vi "Activate-combined-measurement-hardware.vi"(8 "error in (no error)":errorcluster, 11 "SM1000-control in":T1) -> (0 "error out":errorcluster, 1 "Signals":refnum<k21>, 2 "Control":refnum<k21>, 3 "SM1000-control out":T1, 4 "Batch size":i32)   [LabVIEW 2013, in "MaterialCharacterization.lvlib" / "MC-SM1000.lvclass"]
uses:
  MC-SM1000.lvclass
  Object-reference.ctl
  MC-SM1000.lvclass/MC-SM1000.ctl
  <vilib>/DAQmx/create/channels.llb/DAQmx Create Channel (DI-Digital Input).vi
  <vilib>/DAQmx/configure/timing.llb/DAQmx Timing (Sample Clock).vi
  <vilib>/DAQmx/create/channels.llb/DAQmx Create Channel (AI-Temperature-Thermocouple).vi
  <vilib>/DAQmx/create/channels.llb/DAQmx Create Channel (AI-Voltage-Basic).vi
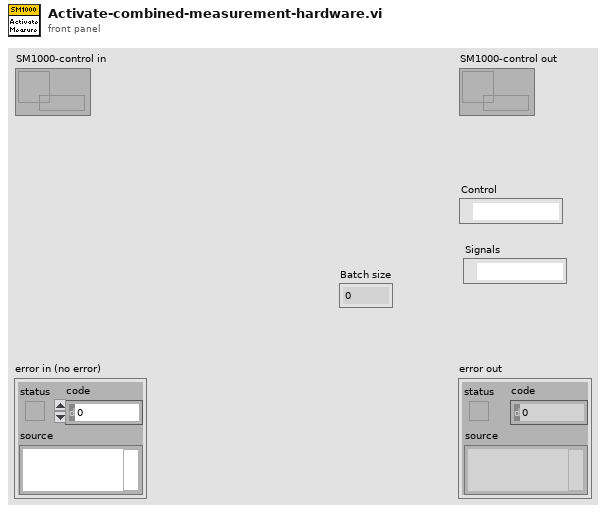
[diagram p1: front panel]
types:
  T1 = typedef "MaterialCharacterization.lvlib/MC-SM1000.lvclass/Object-reference.ctl" = refnum<data-value>
  T2 = typedef "MaterialCharacterization.lvlib/MC-SM1000.lvclass/Combined-settings.ctl" = cluster{"Sample rate":dbl, "Batch size":i32, "Modulation channel":tag, "Temperature channel":tag, "Reflection channel":tag, "Power channel":tag}
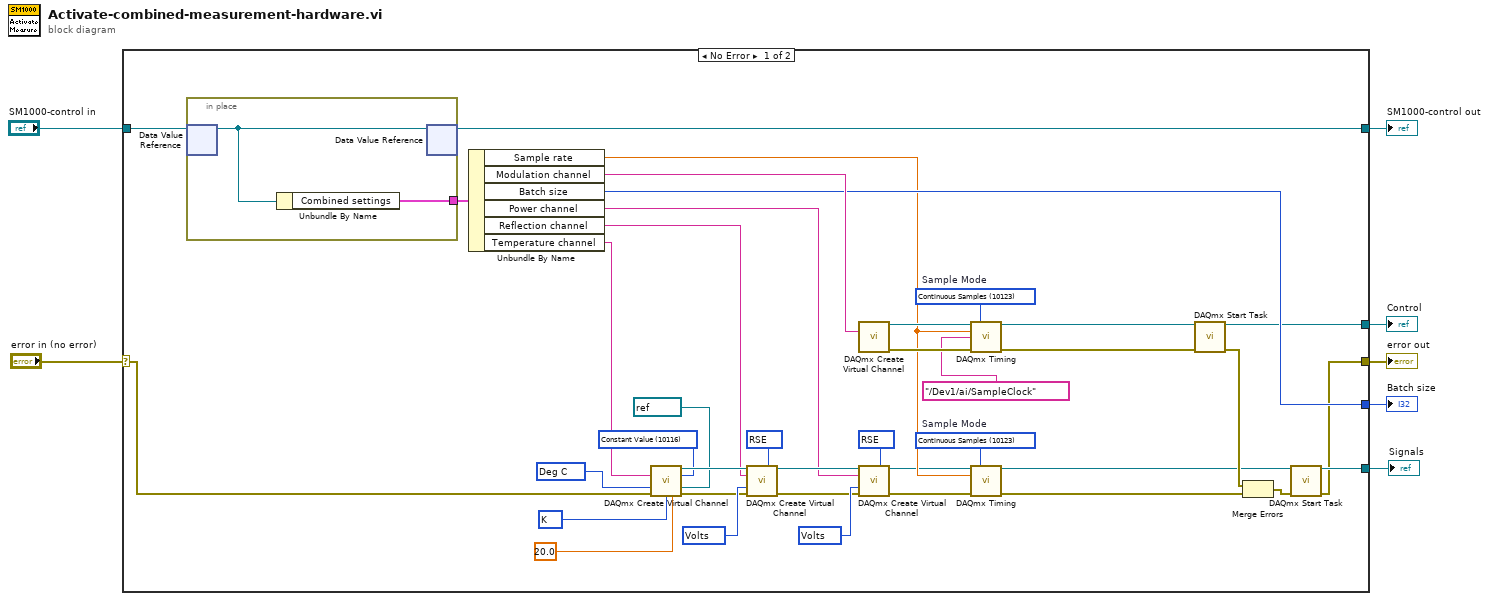
[diagram p0: block diagram]
diagram:
  n1 = case shown="No Error" "error in (no error)" {
    selector: "error in (no error)" -> [w16 w50]
    tunnel: [w32 w50] -> w6
    tunnel: [w45 w49] -> w4
    tunnel: "SM1000-control in" -> [w46 w49]
    tunnel: [w31 _] -> w3
    tunnel: [w39 _] -> w2
    tunnel: [w35 _] -> w1
    frame No Error {
      w11 = 10143 items=["Deg C"=10143, "Deg F"=10144, "Kelvins"=10325, "Deg R"=10145, "From Custom Scale"=10065] ("units")
      w13 = 10116 items=["Built-In"=10200, "Constant Value"=10116, "Channel"=10113] ("cjc source")
      w15 = 10073 items=["J"=10072, "K"=10073, "N"=10077, "R"=10082, "S"=10085, "T"=10086, "B"=10047, "E"=10055] ("thermocouple type")
      w25 = 10348 items=["Volts"=10348, "From Custom Scale"=10065] ("units")
      w24 = 10083 items=["default"=-1, "RSE"=10083, "NRSE"=10078, "Differential"=10106, "Pseudodifferential"=12529] ("input terminal configuration")
      w36 = 10348 items=["Volts"=10348, "From Custom Scale"=10065] ("units")
      w37 = 10083 items=["default"=-1, "RSE"=10083, "NRSE"=10078, "Differential"=10106, "Pseudodifferential"=12529] ("input terminal configuration")
      w38 = 10123 items=["Finite Samples"=10178, "Continuous Samples"=10123, "Hardware Timed Single Point"=12522]  # Sample Mode
      w43 = 10123 items=["Finite Samples"=10178, "Continuous Samples"=10123, "Hardware Timed Single Point"=12522]  # Sample Mode
      n2 = in-place {
        in-place-border: [w47] -> w44
        n3 = in-place-dvr #1(w46) -> (w48:refnum<class "MC-SM1000.lvclass">)  [unwired: 1 out]
        n4 = Unbundle By Name(w48) -> ("Combined settings"=w47:T2)
        n5 = in-place-dvr #1(w48) -> (w45:T1)  [unwired: 1 out]
      }
      n6 = Unbundle By Name(w44) -> ("Sample rate"=w26:dbl, "Modulation channel"=w40:tag, "Batch size"=w39:i32, "Power channel"=w9:tag, "Reflection channel"=w10:tag, "Temperature channel"=w12:tag)
      n7 = call-poly <vilib>:"DAQmx Create Virtual Channel.vi"("physical channels"=w12, "cjc source"=w13, "units"=w11, "cjc channel"=refnum<k21> "CJC", "error in"=w16, "thermocouple type"=w15, "cjc value"=20.0) -> ("task out"=w18:refnum<k21>, "error out"=w17:errorcluster)  [unwired: 7 in]
      n8 = call-poly <vilib>:"DAQmx Create Virtual Channel.vi"("task in"=w18, "input terminal configuration"=w37, "physical channels"=w10, "units"=w36, "error in"=w17) -> ("task out"=w23:refnum<k21>, "error out"=w19:errorcluster)  [unwired: 9 in]
      n9 = call-poly <vilib>:"DAQmx Create Virtual Channel.vi"("lines"=w40) -> ("task out"=w42:refnum<k21>, "error out"=w41:errorcluster)  [unwired: 13 in]
      n10 = call-poly <vilib>:"DAQmx Create Virtual Channel.vi"("task in"=w23, "input terminal configuration"=w24, "physical channels"=w9, "units"=w25, "error in"=w19) -> ("task out"=w22:refnum<k21>, "error out"=w21:errorcluster)  [unwired: 9 in]
      n11 = call-poly <vilib>:"DAQmx Timing.vi"("task/channels in"=w42, "sample mode"=w43, "rate"=w26, "source"=tag "/Dev1/ai/SampleClock", "error in"=w41) -> ("task out"=w27:refnum<k21>, "error out"=w20:errorcluster)  [unwired: 9 in]
      n12 = call-poly <vilib>:"DAQmx Timing.vi"("task/channels in"=w22, "sample mode"=w38, "rate"=w26, "error in"=w21) -> ("task out"=w29:refnum<k21>, "error out"=w28:errorcluster)  [unwired: 10 in]
      n13 = call <vilib>:"DAQmx Start Task.vi"("task/channels in"=w27, "error in"=w20) -> ("task out"=w31:refnum<k21>, "error out"=w33:errorcluster)  [unwired: 12 in]
      n14 = Merge Errors(w33, w28) -> (w34:errorcluster)
      n15 = call <vilib>:"DAQmx Start Task.vi"("task/channels in"=w29, "error in"=w34) -> ("task out"=w35:refnum<k21>, "error out"=w32:errorcluster)  [unwired: 12 in]
    }
    frame Error {
    }
  }
  "error out" <- w6
  "SM1000-control out" <- w4
  "Control" <- w3
  "Batch size" <- w2
  "Signals" <- w1
